vi "StringSplitter.vi"(1 "Input String":string="FPSP0RP0FS0TL0PP50%TD1000FEBL1CL0RL1FL0AL1HL1G3") -> (14 "S0":string, 15 "S1":string, 16 "S2":string, 17 "S3":string, 18 "S4":string, 19 "S5":string)   [LabVIEW 2014]
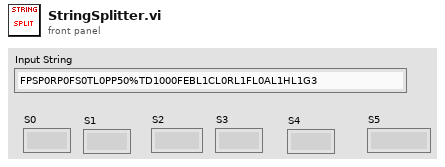
[diagram p1: front panel]
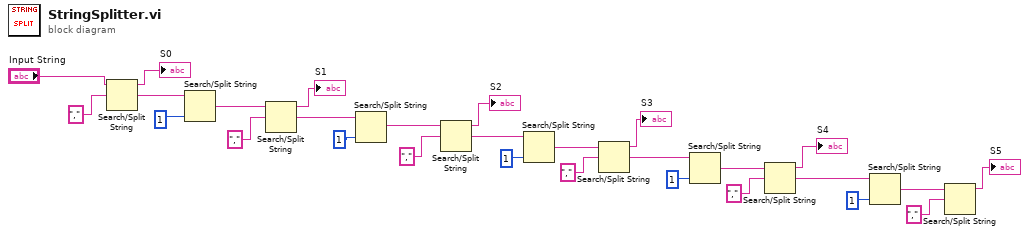
[diagram p0: block diagram]
diagram:
  n1 = Search/Split String(string="Input String", search string/char (-)=",") -> (substring before match=→"S0":string, match + rest of string=w3:string)  [unwired: 1 in, 1 out]
  n2 = Search/Split String(string=w3, offset (0)=1) -> (match + rest of string=w2:string)  [unwired: 1 in, 2 out]
  n3 = Search/Split String(string=w2, search string/char (-)=",") -> (substring before match=→"S1":string, match + rest of string=w4:string)  [unwired: 1 in, 1 out]
  n4 = Search/Split String(string=w4, offset (0)=1) -> (match + rest of string=w5:string)  [unwired: 1 in, 2 out]
  n5 = Search/Split String(string=w5, search string/char (-)=",") -> (substring before match=→"S2":string, match + rest of string=w21:string)  [unwired: 1 in, 1 out]
  n6 = Search/Split String(string=w21, offset (0)=1) -> (match + rest of string=w19:string)  [unwired: 1 in, 2 out]
  n7 = Search/Split String(string=w19, search string/char (-)=",") -> (substring before match=→"S3":string, match + rest of string=w13:string)  [unwired: 1 in, 1 out]
  n8 = Search/Split String(string=w13, offset (0)=1) -> (match + rest of string=w15:string)  [unwired: 1 in, 2 out]
  n9 = Search/Split String(string=w15, search string/char (-)=",") -> (substring before match=→"S4":string, match + rest of string=w8:string)  [unwired: 1 in, 1 out]
  n10 = Search/Split String(string=w8, offset (0)=1) -> (match + rest of string=w10:string)  [unwired: 1 in, 2 out]
  n11 = Search/Split String(string=w10, search string/char (-)=",") -> (substring before match=→"S5":string)  [unwired: 1 in, 2 out]
